vi "com port send data return response.vi"(7 "Return line number":u32, 8 "error in (no error)":errorcluster, 9 "Wait Msecs for response":dbl=1000.0, 10 "Send data":string, 11 "VISA resource name":refnum<visa-resource-name>) -> (0 "error out":errorcluster, 1 "return count":u32, 2 "response":string, 3 "VISA resource name out":refnum<visa-resource-name>, 5 "Response Line":string)   [LabVIEW 2024]
uses:
  <vilib>/Utility/error.llb/whitespace.ctl
  <vilib>/Utility/error.llb/Trim Whitespace One-Sided.vi
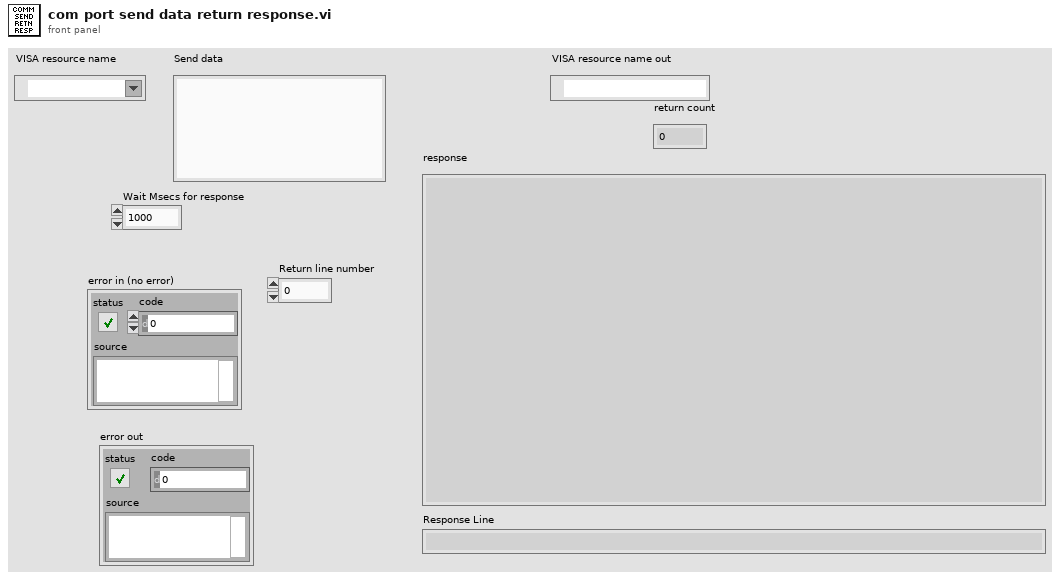
[diagram p1: front panel]
types:
  T1 = typedef "whitespace.ctl" = u16
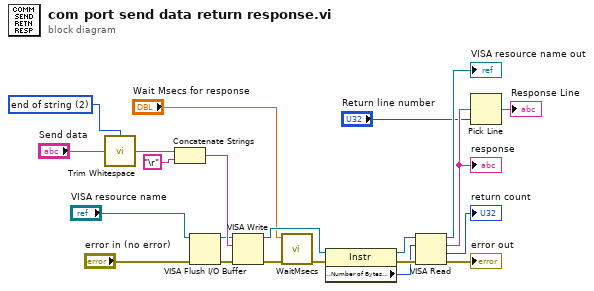
[diagram p0: block diagram]
diagram:
  w12 = T1 2 items=["both", "start of string", "end of string"] ("location (both)")
  n1 = call <vilib>:"Trim Whitespace.vi"("string"="Send data", "location (both)"=w12) -> ("trimmed string"=w10:string)
  n2 = Concatenate Strings(w10, "\r") -> (w8:string)
  n3 = VISA Flush I/O Buffer(VISA resource name="VISA resource name", error in (no error)="error in (no error)") -> (VISA resource name out=w4:refnum<visa-resource-name>, error out=w6:errorcluster)  [unwired: 1 in]
  n4 = VISA Write(VISA resource name=w4, write buffer=w8, error in (no error)=w6) -> (VISA resource name out=w21:refnum<visa-resource-name>, error out=w22:errorcluster)  [unwired: 1 out]
  n5 = call "WaitMsecs.vi"("error in (no error)"=w22, "Wait Msecs"="Wait Msecs for response") -> ("error out"=w20:errorcluster)  [unwired: 9 in]
  n6 = property class="Instr"(reference=w21, error in=w20) -> (reference out=w18:refnum<visa-resource-name>, error out=w19:errorcluster, "Serial Settings:Number of Bytes at Serial Port"=w17:u32)
  n7 = VISA Read(VISA resource name=w18, byte count=w17, error in (no error)=w19) -> (VISA resource name out=→"VISA resource name out":refnum<visa-resource-name>, read buffer=w3:string, return count=→"return count":u32, error out=→"error out":errorcluster)
  "response" <- w3
  n8 = Pick Line(multi-line string=w3, line index="Return line number") -> (output string=→"Response Line":string)  [unwired: 1 in]
